vi "WritePortStatus.vi"(8 "error in (no error)":errorcluster, 9 "Value":string, 10 "Port":dbl, 11 "Cypress in":refnum<class "Cypress.lvclass">) -> (0 "error out":errorcluster, 3 "Cypress out":refnum<class "Cypress.lvclass">)   [LabVIEW 2020, in "Cypress.lvclass"]
uses:
  Cypress.lvclass
  Cypress.lvclass/Cypress.ctl
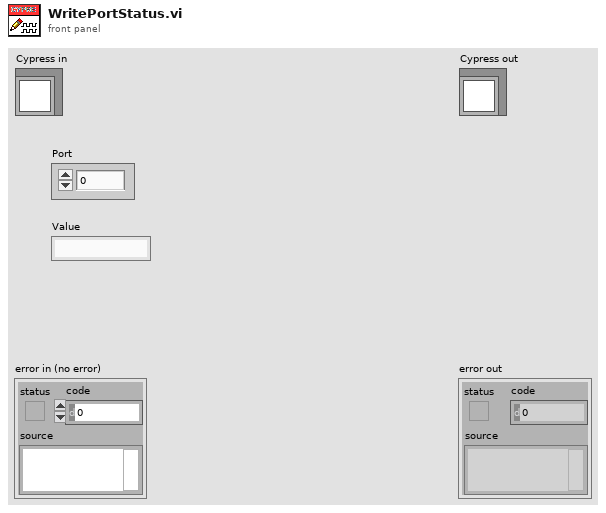
[diagram p1: front panel]
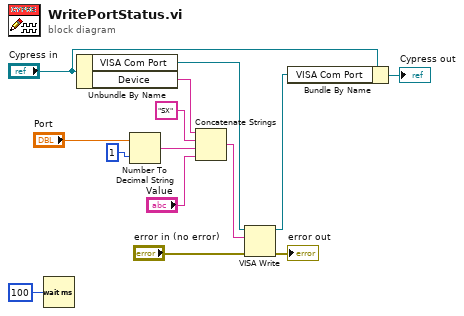
[diagram p0: block diagram]
diagram:
  n1 = Wait (ms)(milliseconds to wait=u32 100) -> ()  [unwired: 1 out]
  n2 = Unbundle By Name("Cypress in") -> ("VISA Com Port"=w9:refnum<visa-resource-name>, "Device"=w8:string)
  n3 = Number To Decimal String(number="Port", width (-)=i16 1) -> (decimal integer string=w12:string)
  n4 = Concatenate Strings(w8, "SX" ("string"), w12, "Value") -> (w14:string)
  n5 = VISA Write(VISA resource name=w9, write buffer=w14, error in (no error)="error in (no error)") -> (VISA resource name out=w11:refnum<visa-resource-name>, error out=→"error out":errorcluster)  [unwired: 1 out]
  n6 = Bundle By Name(cluster="Cypress in", "VISA Com Port"=w11) -> (→"Cypress out":refnum<class "Cypress.lvclass">)
